vi "rad_ConvertImageFiles.vi"(4 "error in":errorcluster, 5 "ImageFiles":string[](array[string]), 7 "ImageFolderRoot":path) -> (0 "error out":errorcluster)   [LabVIEW 2013]
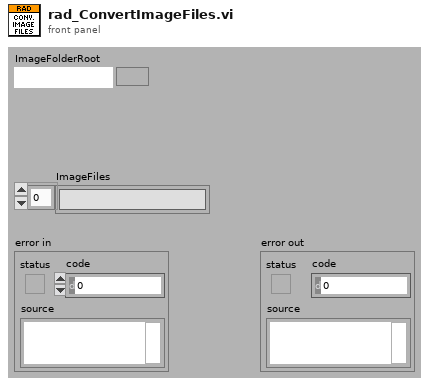
[diagram p1: front panel]
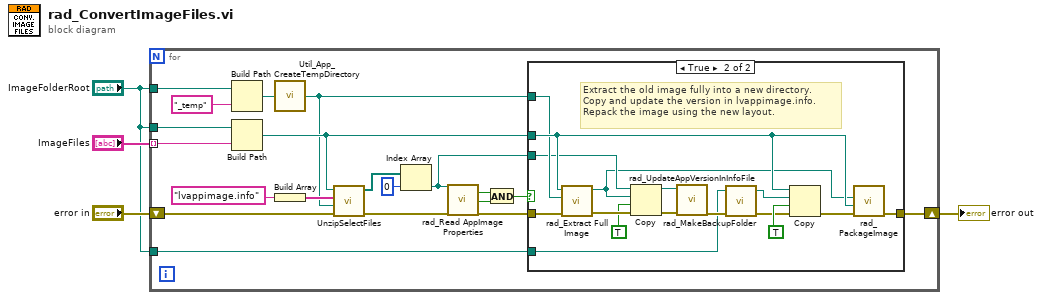
[diagram p0: block diagram]
diagram:
  n1 = for {
    tunnel: "ImageFiles" -> [w15] mode=indexing
    tunnel: "ImageFolderRoot" -> [w23]
    tunnel: "ImageFolderRoot" -> [w19]
    shift-right: [w18] -> w4
    shift-left: "error in" -> [w10]
    tunnel: "ImageFolderRoot" -> [w16]
    n2 = Build Path(base path=w23, name or relative path="_temp") -> (appended path=w17:path)
    n3 = Build Path(base path=w16, name or relative path=w15) -> (appended path=w14:path)
    n4 = call "Util_App_CreateTempDirectory.vi"("TempFolderPath"=w17) -> ("TempFolderPath_out"=w11:path)
    n5 = Build Array("lvappimage.info") -> (w12:string[])
    n6 = call "UnzipSelectFiles.vi"("error in (no error)"=w10, "Target directory (same as Zip file if empty)"=w11, "Files to Unzip"=w12, "Zip file"=w14) -> ("error out"=w8:errorcluster, "Unzipped files"=w7:path[])  [unwired: 5 in, 1 out]
    n7 = Index Array(array=w7, index=0) -> (element=w5:path)
    n8 = call "rad_Read AppImage Properties.vi"("AppImage Properties Path"=w5, "error in (no error)"=w8) -> ("Supported"=w22:bool, "Older"=w21:bool, "error out"=w9:errorcluster)  [unwired: 12 in, 3 out]
    n9 = And(x=w22, y=w21) -> (x .and. y?=w20:bool)
    n10 = case shown="True" w20 {
      tunnel: w14 -> [_ w33]
      tunnel: w11 -> [_ w32]
      tunnel: w19 -> [_ w37]
      tunnel: [w25 w35] -> w18
      tunnel: w9 -> [w25 w34]
      tunnel: w5 -> [_ w29]
      frame False {
      }
      frame True {
        # "Extract the old image fully into a new directory.\nCopy and update the version in lvappimage.info.\nRepack the image using the new layout."
        n11 = call "rad_Extract Full Image.vi"("error in (no error)"=w34, "App Image Temp Folder"=w32, "Zipped App Image File Path"=w33) -> ("error out"=w31:errorcluster, "Unzipped App Image Folder Path"=w28:path)  [unwired: 7 in]
        n12 = Copy(8:w31, 9:TRUE ("overwrite (F)"), 10:w28, 11:w29) -> (0:w30:errorcluster, 3:w27:path)  [unwired: 1 in, 1 out]
        n13 = call "rad_UpdateAppVersionInInfoFile.vi"("error in"=w30, "Path to lvappimage.info"=w27) -> ("error out"=w40:errorcluster)  [unwired: 9 in]
        n14 = call "rad_MakeBackupFolder.vi"("error in"=w40, "ImagePathFolder"=w37) -> ("error out"=w39:errorcluster, "BackupFolderPath"=w38:path)  [unwired: 2 in]
        n15 = Copy(8:w39, 9:TRUE ("overwrite (F)"), 10:w38, 11:w33) -> (0:w36:errorcluster)  [unwired: 1 in, 2 out]
        n16 = call "rad_PackageImage.vi"("error in (no error)"=w36, "AppImage Path"=w33, "Temp Image Path"=w28) -> ("error out"=w35:errorcluster)  [unwired: 8 in]
      }
    }
  }
  "error out" <- w4
